vi "Step1_21_LowPass.vi"(9 "s_axis_data_tdata":fxp<+/-,16,1>, 10 "s_axis_data_tvalid":bool) -> (1 "m_axis_data_tdata":fxp<+/-,24,1>, 2 "m_axis_data_tvalid":bool, 3 "s_axis_data_tready":bool)   [LabVIEW 2018]
uses:
  <vilib>/rvi/XilinxIP/XIPIN_XNode/niFpgaXIPIN.xnode
  Deprecated_Delete/DigitalFilterDesign/FIR_Filter_Configuration/FIR Compiler/xsim.dir/FIR_Compiler_3CE652926F5B43F18022D1349C670FA0/xsimk_3CE652926F5B43F18022D1349C670FA0.dll
  <vilib>/rvi/IPIntegrationNode/IPINode_Xnode/niFpgaIPINode.xnode
  <vilib>/rvi/IPIntegrationNode/IPINode_Typedef/niFpgaIPINodeSupportedFamilies.ctl
  <vilib>/rvi/IPIntegrationNode/IPINode_Utilities/niFpgaIPINodeSimCore.vi
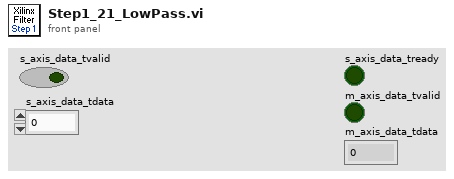
[diagram p1: front panel]
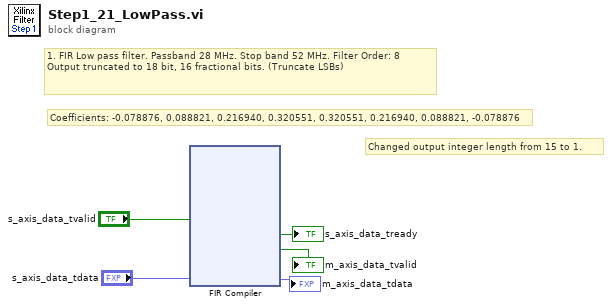
[diagram p0: block diagram]
diagram:
  # "Changed output integer length from 15 to 1."
  # "Coefficients: -0.078876, 0.088821, 0.216940, 0.320551, 0.320551, 0.216940, 0.088821, -0.078876"
  # "1.\tFIR Low pass filter. Passband 28 MHz. Stop band 52 MHz. Filter Order: 8 \nOutput truncated to 18 bit, 16 fractional bits. (Truncate LSBs)"
  n1 = xnode ("FIR Compiler")("s_axis_data_tvalid"="s_axis_data_tvalid", "s_axis_data_tdata"="s_axis_data_tdata") -> ("s_axis_data_tready"=→"s_axis_data_tready":bool, "m_axis_data_tvalid"=→"m_axis_data_tvalid":bool, "m_axis_data_tdata"=→"m_axis_data_tdata":fxp<+/-,24,1>)
